vi "Check For Colour.vi"(0 "Image":T2(plugin-control)=refnum, 1 "Colour Definition":T1={"Hue Range"={"Lower value"=5, "Upper value"=255}, "Saturation Range"={"Lower value"=100, "Upper value"=255}, "Luminosity Range"={"Lower value"=100, "Upper value"=255}}) -> (7 "Proportion":dbl=99.0)   [LabVIEW 2017]
uses:
  <vilib>/vision/NI_Vision_Development_Module.lvlib
panel:
  out "error out":errorcluster
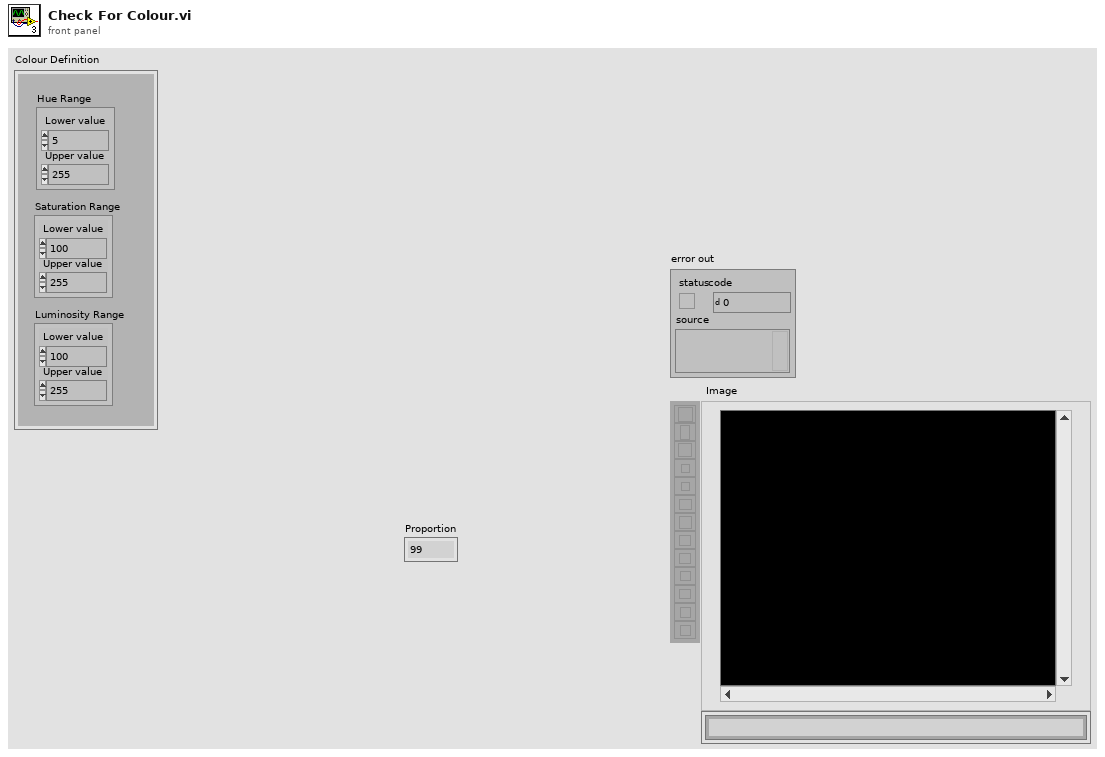
[diagram p1: front panel]
types:
  T1 = cluster{"Hue Range":cluster{"Lower value":i32, "Upper value":i32}, "Saturation Range":cluster{"Lower value":i32, "Upper value":i32}, "Luminosity Range":cluster{"Lower value":i32, "Upper value":i32}}
  T2 = typedef "IMAQ Image.ctl" = refnum<image>
  T3 = typedef "Image Type" = u32
  T4 = cluster{"histogram":u32[], "Minimal Value":sgl, "Maximal Value":sgl, "Starting Value":sgl, "Interval Width":sgl, "Mean Value":sgl, "Standard  Variation":sgl, "Area (pixels)":i32}
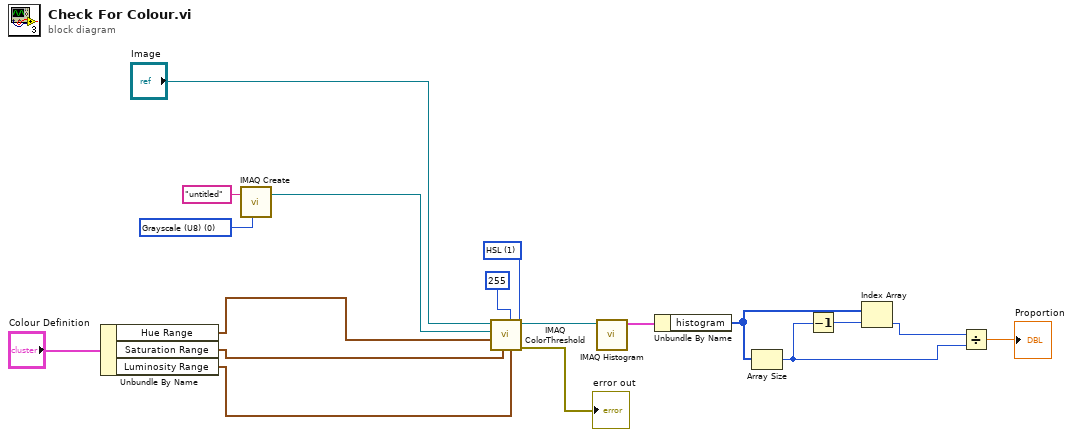
[diagram p0: block diagram]
diagram:
  w11 = T3 0 items=["Grayscale (U8)", "Grayscale (I16)", "Grayscale (SGL)", "Complex (CSG)", "RGB (U32)", "HSL (U32)", "RGB (U64)", "Grayscale (U16)"] ("Image Type")
  w16 = u16 1 items=["RGB", "HSL", "HSV", "HSI"] ("Color Mode")
  n1 = Unbundle By Name("Colour Definition") -> ("Hue Range"=w3:cluster{"Lower value":i32, "Upper value":i32}, "Saturation Range"=w2:cluster{"Lower value":i32, "Upper value":i32}, "Luminosity Range"=w1:cluster{"Lower value":i32, "Upper value":i32})
  n2 = call "IMAQ Create"("Image Name"="untitled", "Image Type"=w11) -> ("New Image"=w10:T2)  [unwired: 3 in, 1 out]
  n3 = call "IMAQ ColorThreshold"("Blue or Luma or Val or Inten Range"=w1, "Replace Value"=255, "Green or Sat Range"=w2, "Color Mode"=w16, "Red or Hue Range"=w3, "Image Dst"=w10, "Image Src"="Image") -> ("error out"=→"error out":errorcluster, "Image Dst Out"=w9:T2)  [unwired: 1 in, 2 out]
  n4 = call "IMAQ Histogram"("Image"=w9) -> ("Histogram Report"=w13:T4)  [unwired: 9 in, 1 out]
  n5 = Unbundle By Name(w13) -> ("histogram"=w8:u32[])
  n6 = Array Size(array=w8) -> (size(s)=w7:i32)
  n7 = Decrement(x=w7) -> (x-1=w6:i32)
  n8 = Index Array(array=w8, index=w6) -> (element=w5:u32)
  n9 = Divide(x=w5, y=w7) -> (x/y=→"Proportion":dbl)
